vi "Close Vecto.vi"(8 "error in (no error)":errorcluster, 11 "VolatusCoreTask in":refnum<class "VolatusCoreTask.lvclass">) -> (0 "error out":errorcluster, 3 "VolatusCoreTask out":refnum<class "VolatusCoreTask.lvclass">)   [LabVIEW 2020, in "Volatus.lvlib" / "VolatusCoreTask.lvclass"]
uses:
  VolatusCoreTask.lvclass
  VolatusCoreTask.lvclass/VolatusCoreTask.ctl
  lv-vecto/Vecto/Vecto/Vecto.lvclass
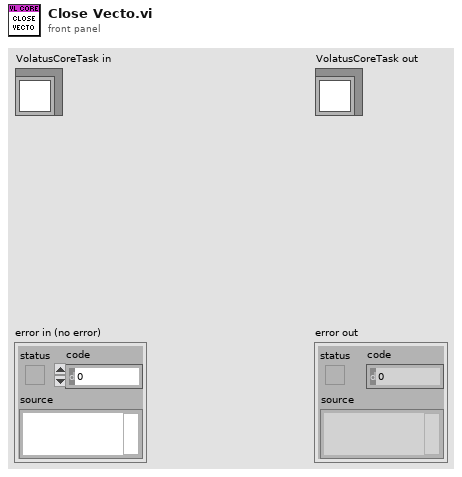
[diagram p1: front panel]
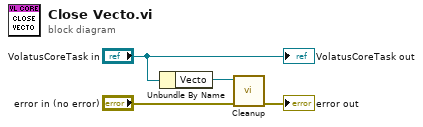
[diagram p0: block diagram]
diagram:
  n1 = Unbundle By Name("VolatusCoreTask in") -> ("Vecto"=w3:refnum<class "Vecto.lvclass">)
  n2 = call "Cleanup.vi"("error in (no error)"="error in (no error)", "Vecto in"=w3) -> ("error out"=→"error out":errorcluster)  [unwired: 9 in]
  "VolatusCoreTask out" <- "VolatusCoreTask in"
